vi "Exit Application.vi"(0 "exit? (T)":bool=TRUE, 5 "exit code":i32, 11 "error in (no error)":errorcluster) -> (15 "error out":errorcluster)   [LabVIEW 2015, in "LV System Utils v1.lvlib"]
doc: "Exits LabVIEW if application works in Run Time System, otherwise stops the application.\n\nIf error code is other than 0, application will terminate immediately, which means that LabVIEW will not have a chance to do the regular clean-up (closing file handles, removing temporary files etc.)."
uses:
  <userlib>/LV System Utils v1/LV System Utils v1.lvlib
  Windows/System32/msvcrt.dll
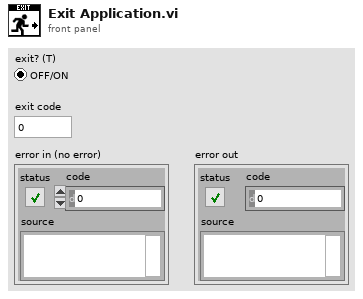
[diagram p1: front panel]
types:
  T1 = enum32{"invalid app kind", "Development System", "Run Time System", "Student Edition", "Embedded LabVIEW", "Evaluation", "Custom"}
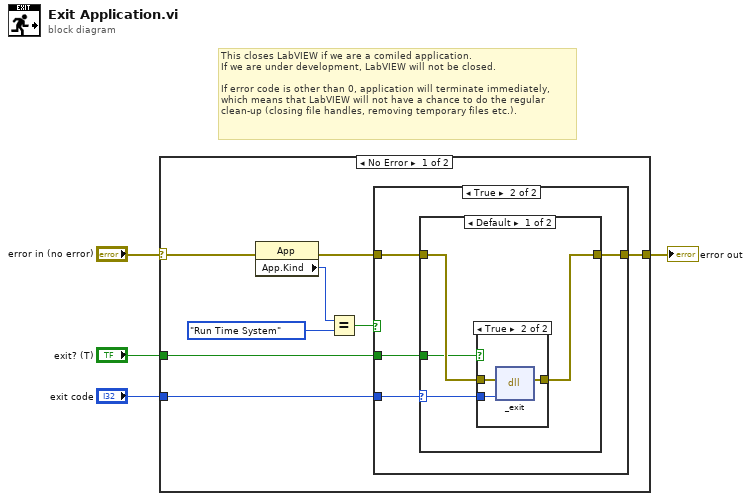
[diagram p0: block diagram]
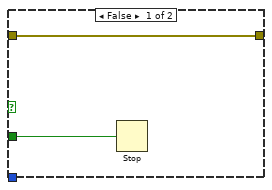
[diagram p2: hidden frame]
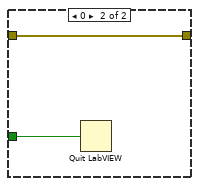
[diagram p4: hidden frame]
diagram:
  # "This closes LabVIEW if we are a comiled application.\nIf we are under development, LabVIEW will not be closed.\n\nIf error code is other than 0, application will terminate immediately,\nwhich means that LabVIEW will not have a chance to do the regular\nclean-up (closing file handles, removing temporary files etc.)."
  n1 = case shown="No Error" "error in (no error)" {
    selector: "error in (no error)" -> [w5 w29]
    tunnel: "exit? (T)" -> [w9 _]
    tunnel: "exit code" -> [w8 _]
    tunnel: [w6 w29] -> w2
    frame No Error {
      n2 = property class="App"(error in=w5) -> (error out=w7:errorcluster, "App.Kind"=w12:T1)  [unwired: 1 in, 1 out]
      n3 = Equal?(x=w12, y=T1."Run Time System" ("Application:Kind")) -> (x = y?=w10:bool)
      n4 = case shown="True" w10 {
        tunnel: w9 -> [w14 w18]
        tunnel: w8 -> [_ w17]
        tunnel: w7 -> [w13 w16]
        tunnel: [w13 w15] -> w6
        frame False {
          n5 = Stop(stop? (T)=w14) -> ()
        }
        frame True {
          n6 = case shown="Default" w17 {
            selector: w17 -> [w20 _]
            tunnel: w18 -> [w19 w28]
            tunnel: w16 -> [w22 w27]
            tunnel: [w21 w27] -> w15
            frame Default {
              n7 = case shown="True" w19 {
                tunnel: w22 -> [w23 w26]
                tunnel: [w23 w25] -> w21
                tunnel: w20 -> [_ w24]
                frame False {
                }
                frame True {
                  n8 = dll-call lib="C:/Windows/System32/msvcrt.dll" fn="_exit"(error in=w26, "code"=w24) -> (error out=w25:errorcluster)  [unwired: 4 in, 1 out]
                }
              }
            }
            frame 0 {
              n9 = Quit LabVIEW(quit? (T)=w28) -> ()
            }
          }
        }
      }
    }
    frame Error {
    }
  }
  "error out" <- w2
